vi "检查曲线文件.vi"(8 "Error In":errorcluster, 11 "Folder Path":path caption="文件夹路径") -> (0 "Error Out":errorcluster, 1 "All Files in Dir":path[](array[path]) caption="目录中的所有文件", 2 "Exit?":bool, 3 "曲线文件路径":path)   [LabVIEW 2018]
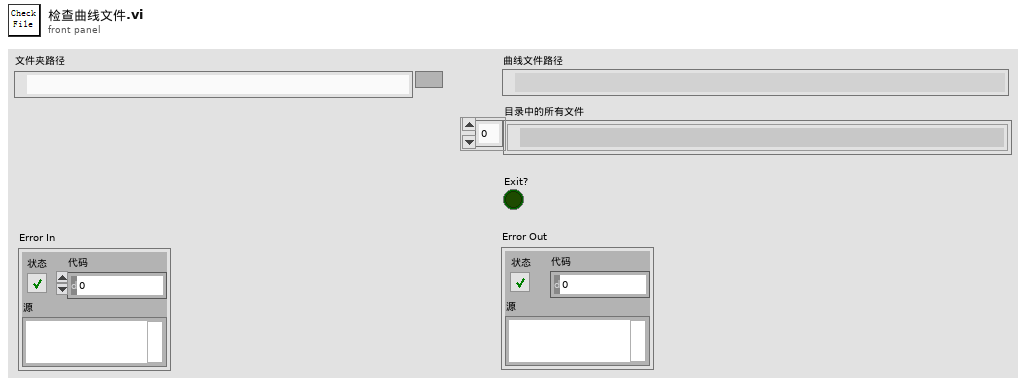
[diagram p1: front panel]
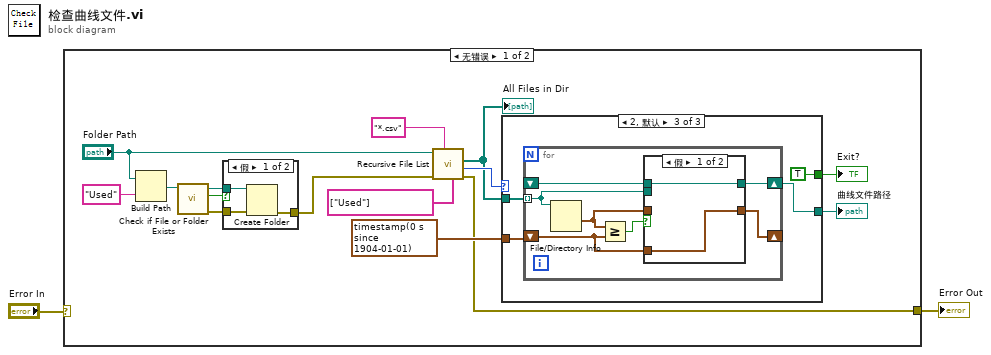
[diagram p0: block diagram]
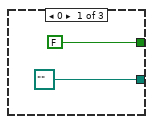
[diagram p3: hidden frame]
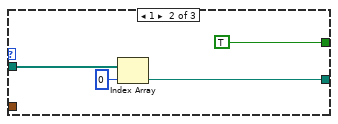
[diagram p4: hidden frame]
diagram:
  n1 = case shown="无错误" "Error In" {
    selector: "Error In" -> [_ w43]
    tunnel: [w11 w43] -> w1
    frame No Error {
      n2 = Build Path(base path="Folder Path", name or relative path="Used" ("名称或相对路径")) -> (appended path=w8:path)
      n3 = call <vilib>:"Check if File or Folder Exists.vi"("path"=w8) -> ("error out"=w5:errorcluster, "file or folder exists?"=w7:bool, "dup path"=w6:path)  [unwired: 8 in]
      n4 = case shown="假" w7 {
        tunnel: w6 -> [w20 _]
        tunnel: w5 -> [w19 w21]
        tunnel: [w18 w21] -> w4
        frame False {
          n5 = Create Folder(path (use dialog)=w20, error in=w19) -> (error out=w18:errorcluster)  [unwired: 1 in, 2 out]
        }
        frame True {
        }
      }
      n6 = call <vilib>:"Recursive File List.vi"("Folders to Exclude"=string[] ["Used"], "pattern"="*.csv", "error in (no error)"=w4, "Folder Path"="Folder Path") -> ("error out"=w11:errorcluster, "Number of Files"=w16:i32, "All Files in Dir"=w15:path[])  [unwired: 3 in, 2 out]
      "All Files in Dir" <- w15
      n7 = case shown="2, 默认" w16 {
        tunnel: w15 -> [_ w27 w31]
        tunnel: [path "" w25 w29] -> w14
        tunnel: [FALSE TRUE TRUE] -> w13
        tunnel: timestamp(0 s since 1904-01-01) ("上次修改 2") -> [_ _ w30]
        frame 0 {
        }
        frame 1 {
          n8 = Index Array(array=w27, index=0 ("索引")) -> (element=w25:path)
        }
        frame 2, Default {
          n9 = for {
            tunnel: w31 -> [w35] mode=indexing
            shift-right: [w33] -> _
            shift-left: w30 -> [w32]
            shift-right: [w37] -> w29
            shift-left: _ -> [w36]
            n10 = File/Directory Info(path=w35) -> (last mod=w34:timestamp)  [unwired: 1 in, 6 out]
            n11 = Greater Or Equal?(x=w34, y=w32) -> (x >= y?=w38:bool)
            n12 = case shown="假" w38 {
              tunnel: w36 -> [w40 _]
              tunnel: [w40 w42] -> w37
              tunnel: w35 -> [_ w42]
              tunnel: w34 -> [_ w41]
              tunnel: [w39 w41] -> w33
              tunnel: w32 -> [w39 _]
              frame False {
              }
              frame True {
              }
            }
          }
        }
      }
      "曲线文件路径" <- w14
      "Exit?" <- w13
    }
    frame Error {
    }
  }
  "Error Out" <- w1
